vi "DAQmx Create Channel (CI-Count Edges).vi"(0 "task in":refnum<k21>, 1 "initial count":u32, 2 "count direction":i32(ring)=10128 items=["Count Up"=10128, "Count Down"=10124, "Externally Controlled"=10326], 3 "edge":i32(ring)=10280 items=["Rising"=10280, "Falling"=10171], 5 "counter":tag, 7 "name to assign":string, 11 "error in":errorcluster) -> (4 "task out":refnum<k21>, 15 "error out":errorcluster)   [LabVIEW 2020]
doc: "Creates a channel to count the number of rising or falling edges of a digital signal. With the exception of devices that support multi-counter tasks, you can create only one counter input channel at a time with this VI because a task can contain only one counter input channel. To read from multiple counters simultaneously, use a separate task for each counter. Connect the input signal to the default input terminal of the counter unless you select a different input terminal."
uses:
  nilvaiu.dll
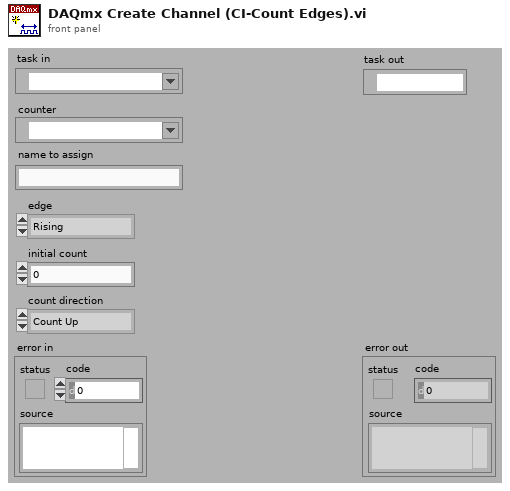
[diagram p1: front panel]
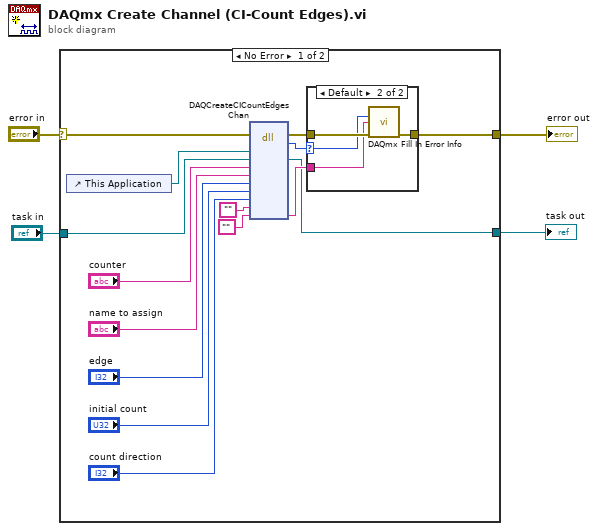
[diagram p0: block diagram]
diagram:
  n1 = case shown="No Error" "error in" {
    selector: "error in" -> [w6 w26]
    tunnel: [w14 w26] -> w4
    tunnel: [w13 w25] -> w3
    tunnel: "task in" -> [w7 w25]
    frame No Error {
      n2 = control-ref of="This Application"() -> (w16:refnum<vi>)
      n3 = dll-call lib="nilvaiu.*" fn="DAQCreateCICountEdgesChan"(error in=w6, "lvAppRef"=w16, "refObjPtr"=w7, "counter"="counter", "channelNameIn"="name to assign", "edge"="edge", "initialCount"="initial count", "direction"="count direction", "channelNamesOut"="", "extendedErrorInfo"="") -> (error out=w19:errorcluster, "return type"=w18:i32, "refObjPtr"=w13:refnum<k21>, "extendedErrorInfo"=w17:string)  [unwired: 9 in, 1 out]
      n4 = case shown="Default" w18 {
        selector: w18 -> [_ w22]
        tunnel: w19 -> [w20 w24]
        tunnel: [w20 w23] -> w14
        tunnel: w17 -> [_ w21]
        frame 0 {
        }
        frame Default {
          n5 = call "DAQmx Fill In Error Info.vi"("status code"=w22, "extended error info"=w21, "error in"=w24) -> ("error out"=w23:errorcluster)  [unwired: 1 in, 11 out]
        }
      }
    }
    frame Error {
    }
  }
  "error out" <- w4
  "task out" <- w3
